vi "Write Available Sensors.vi"(8 "error in (no error)":errorcluster, 10 "Available Sensors":refnum<class "Sensor.lvclass">[](array[class]), 11 "Vessel in":refnum<class "Vessel.lvclass">) -> (0 "error out":errorcluster, 3 "Vessel out":refnum<class "Vessel.lvclass">)   [LabVIEW 2014, in "Vessel.lvclass"]
uses:
  Vessel.lvclass
  Sensor/Sensor.lvclass
  Vessel.lvclass/Vessel.ctl
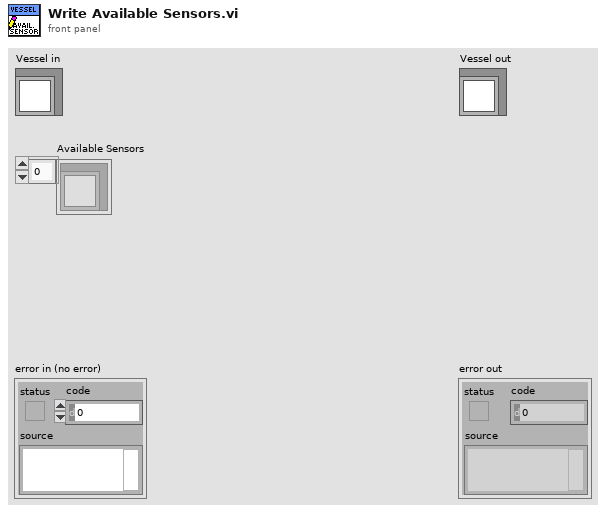
[diagram p1: front panel]
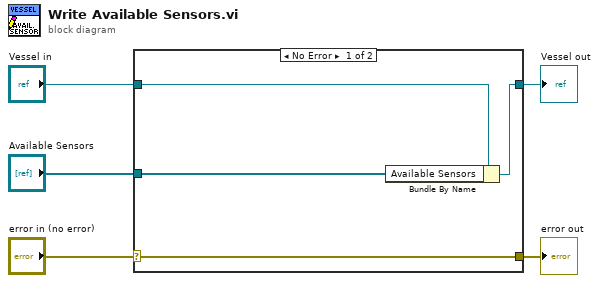
[diagram p0: block diagram]
diagram:
  n1 = case shown="No Error" "error in (no error)" {
    selector: "error in (no error)" -> [w9 w10]
    tunnel: [w9 w10] -> w4
    tunnel: [w7 w11] -> w2
    tunnel: "Vessel in" -> [w8 w11]
    tunnel: "Available Sensors" -> [w6 _]
    frame No Error {
      n2 = Bundle By Name(cluster=w8, "Available Sensors"=w6) -> (w7:refnum<class "Vessel.lvclass">)
    }
    frame Error {
    }
  }
  "error out" <- w4
  "Vessel out" <- w2
